vi "Enable Service Request.vi"(8 "error in (no error)":errorcluster, 10 "Request Enable (0)":i16 min=0 max=255, 11 "VISA resource name":refnum<visa-resource-name>) -> (0 "error out":errorcluster, 3 "VISA resource name out":refnum<visa-resource-name>)   [LabVIEW 2018, in "LTB-1.lvlib" / "3150.lvlib"]
doc: "Sets the status for the Service Request Enable Register bits."
uses:
  3150.lvlib
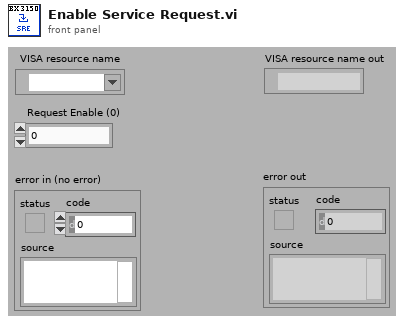
[diagram p1: front panel]
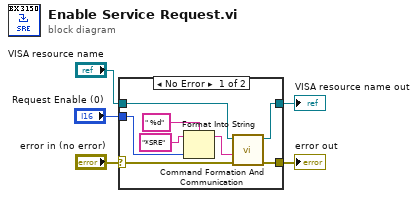
[diagram p0: block diagram]
diagram:
  n1 = case shown="No Error" "error in (no error)" {
    selector: "error in (no error)" -> [w13 w15]
    tunnel: [w12 w15] -> w1
    tunnel: [w11 w14] -> w4
    tunnel: "VISA resource name" -> [w10 w14]
    tunnel: "Request Enable (0)" -> [w8 _]
    frame No Error {
      n2 = Format Into String(format string=" %d", initial string="*SRE" ("Command"), w8) -> (resulting string=w6:string)  [unwired: 1 in, 1 out]
      n3 = call "Command Formation And Communication.vi"("error in (no error)"=w13, "Command"=w6, "VISA resource name"=w10) -> ("error out"=w12:errorcluster, "VISA resource name out"=w11:refnum<visa-resource-name>)  [unwired: 1 in, 6 out]
    }
    frame Error {
    }
  }
  "VISA resource name out" <- w4
  "error out" <- w1
